vi "X轴连续扫描（待完成）.vi"(0 "VISA I":refnum<visa-resource-name>, 3 "X":dbl, 4 "精度":dbl=0.001, 5 "细分设置":dbl=8.0, 6 "等待时间(ms)":u32=40, 7 "pulDDR2Length":u32, 8 "电机急停":bool, 9 "hDevice":i32, 11 "M-length":dbl, 13 "N-length":dbl) -> (14 "VISA O":refnum<visa-resource-name>, 15 "hDevice out":i32, 16 "X":dbl, 17 "强度图行":dbl[](array[numeric]), 18 "时域谱页":dbl[][](array[numeric]), 19 "幅频谱页":dbl[][](array[numeric]))   [LabVIEW 2016]
panel:
  out "大小":i32[](array[numeric])
  out "幅频谱":dbl[](graph)
  out "时域谱":dbl[](graph)
  in  "确定":bool
  in  "ESC":bool
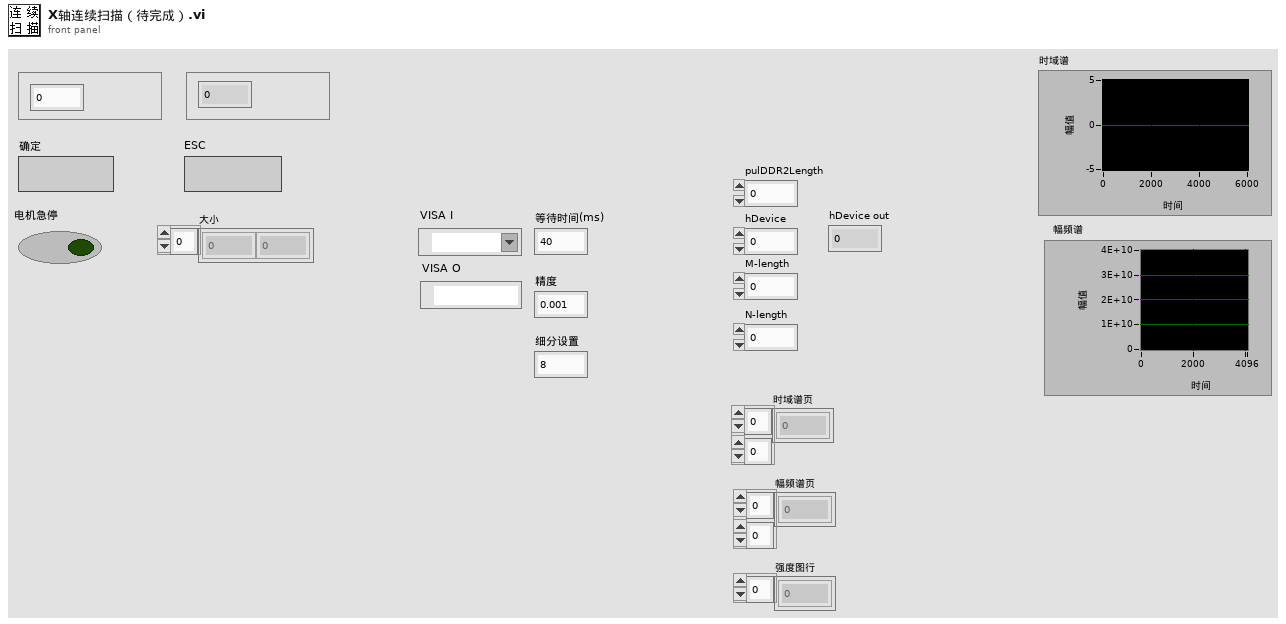
[diagram p1: front panel]
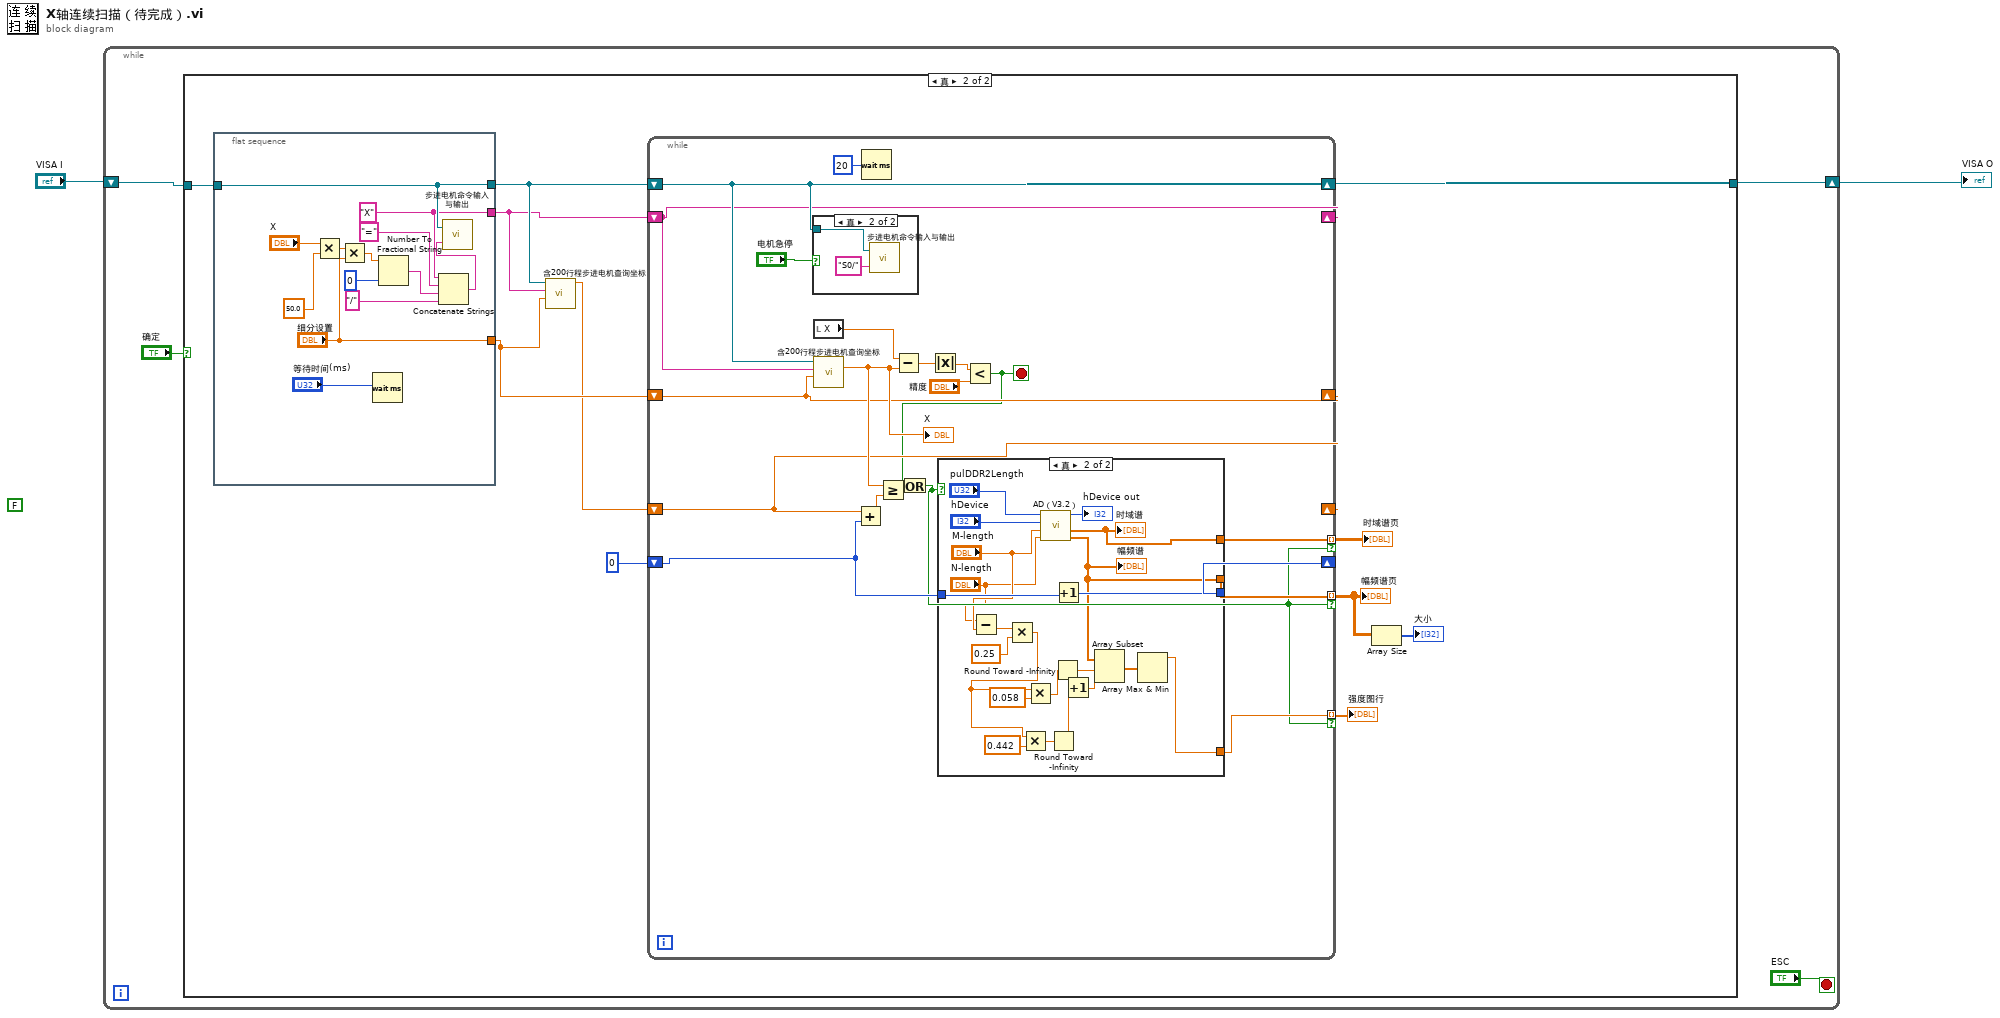
[diagram p0: block diagram]
diagram:
  (unwired) FALSE
  n1 = while {
    shift-right: [w5] -> w2
    shift-left: "VISA I" -> [w6]
    stop <- "ESC" stop-if-true
    n2 = case shown="真" "确定" {
      tunnel: w6 -> [w7 w18]
      tunnel: [w7 w17] -> w5
      frame False {
      }
      frame True {
        n3 = flat-sequence {
          tunnel: w18 -> [w67]
          tunnel: [w67] -> w16
          tunnel: ["细分设置"] -> w14
          tunnel: [w64] -> w15
          frame #0 {
            w64 = "X"
            n4 = Multiply(x="X", y=50.0 ("x")) -> (x*y=w70:dbl)
            n5 = Multiply(x=w70, y="细分设置") -> (x*y=w75:dbl)
            n6 = Wait (ms)(milliseconds to wait="等待时间(ms)") -> ()  [unwired: 1 out]
            n7 = Number To Fractional String(number=w75, precision (6)=i16 0 ("精度(6)")) -> (F-format string=w73:string)  [unwired: 2 out]
            n8 = Concatenate Strings(w64, "=" ("字符串"), w73, "/" ("字符串")) -> (w69:string)
            n9 = call "步进电机命令输入与输出.vi"("输入字符串"=w69, "串口通信端口"=w67) -> ()  [unwired: 1 out]
          }
        }
        n10 = call "含200行程步进电机查询坐标.vi"("细分设置"=w14, "查询坐标轴"=w15, "串口通信端口"=w16) -> ("坐标(mm)"=w13:dbl)  [unwired: 8 in]
        n11 = while {
          shift-right: [w36] -> w17
          shift-left: w16 -> [w36]
          shift-right: [w28] -> _
          shift-left: w13 -> [w28]
          shift-right: [w27] -> _
          shift-left: w14 -> [w27]
          shift-right: [w29] -> _
          shift-left: w15 -> [w29]
          tunnel: [w26] -> w9 mode=indexing if=w20
          shift-right: [w24] -> _
          shift-left: 0 -> [w25]
          tunnel: [w23] -> w11 mode=indexing if=w20
          tunnel: [w22] -> w10 mode=indexing if=w20
          stop <- w19 stop-if-true
          n12 = case shown="真" "电机急停" {
            tunnel: w36 -> [_ w61]
            frame False {
            }
            frame True {
              n13 = call "步进电机命令输入与输出.vi"("输入字符串"="S0/", "串口通信端口"=w61) -> ()  [unwired: 1 out]
            }
          }
          n14 = local read "X"() -> (w32:dbl)
          n15 = call "含200行程步进电机查询坐标.vi"("细分设置"=w27, "查询坐标轴"=w29, "串口通信端口"=w36) -> ("坐标(mm)"=w30:dbl)  [unwired: 8 in]
          "X" <- w30
          n16 = Add(x=w28, y=w25) -> (x+y=w31:dbl)
          n17 = Wait (ms)(milliseconds to wait=u32 20 ("等待时间（毫秒）")) -> ()  [unwired: 1 out]
          n18 = Greater Or Equal?(x=w30, y=w31) -> (x >= y?=w21:bool)
          n19 = Subtract(x=w32, y=w30) -> (x-y=w38:dbl)
          n20 = Absolute Value(x=w38) -> (abs(x)=w37:dbl)
          n21 = Less?(x=w37, y="精度") -> (x < y?=w19:bool)
          n22 = Or(x=w19, y=w21) -> (x .or. y?=w20:bool)
          n23 = case shown="真" w20 {
            tunnel: [_ w41] -> w26
            tunnel: w25 -> [w39 w57]
            tunnel: [w39 w56] -> w24
            tunnel: [_ w55] -> w23
            tunnel: [_ w40] -> w22
            frame False {
            }
            frame True {
              n24 = Subtract(x="N-length", y="M-length") -> (x-y=w53:dbl)
              n25 = Multiply(x=w53, y=0.25) -> (x*y=w43:dbl)
              n26 = Multiply(x=w43, y=0.442) -> (x*y=w46:dbl)
              n27 = Multiply(x=w43, y=0.058) -> (x*y=w48:dbl)
              n28 = call "AD（V3.2）.vi"("N-length"="N-length", "M-length"="M-length", "hDevice"="hDevice", "pulDDR2Length"="pulDDR2Length") -> ("幅频谱"=w41:dbl[], "时域谱"=w55:dbl[], "hDevice out"=→"hDevice out":i32)  [unwired: 5 in]
              "时域谱" <- w55
              "幅频谱" <- w41
              n29 = Round Toward -Infinity(1:w46) -> (0:w44:dbl)
              n30 = Round Toward -Infinity(1:w48) -> (0:w47:dbl)
              n31 = Increment(x=w57) -> (x+1=w56:i32)
              n32 = Increment(x=w44) -> (x+1=w50:dbl)
              n33 = Array Subset(array=w41, index=w47, length=w50) -> (w42:dbl[])
              n34 = Array Max & Min(array=w42) -> (max value=w40:dbl)  [unwired: 3 out]
            }
          }
        }
        "幅频谱页" <- w9
        "时域谱页" <- w11
        "强度图行" <- w10
        n35 = Array Size(array=w9) -> (size(s)=→"大小":i32[])
      }
    }
  }
  "VISA O" <- w2
